vi "Bin to BDC(5-разрядное число).vi"(0 "B":T2) -> (1 "R0":T1, 2 "R1":T1)   [LabVIEW 2013]
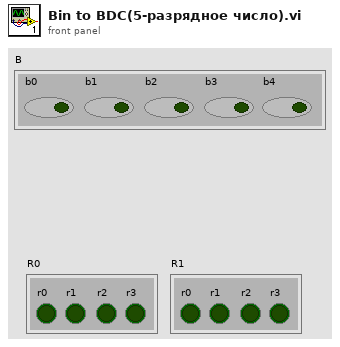
[diagram p1: front panel]
types:
  T1 = cluster{"r0":bool, "r1":bool, "r2":bool, "r3":bool}
  T2 = cluster{"b0":bool, "b1":bool, "b2":bool, "b3":bool, "b4":bool}
  T3 = cluster{"r0":bool, "r1":bool, "r2":bool, "r3":bool, "r4":bool}
  T4 = cluster{"r1":bool, "r2":bool, "r3":bool, "r4":bool}
  T5 = cluster{"d0":bool, "d1":bool, "d2":bool, "d3":bool}
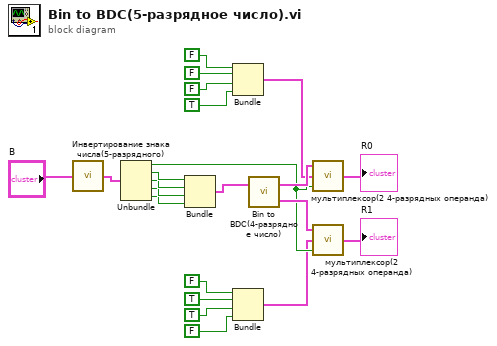
[diagram p0: block diagram]
diagram:
  n1 = call "Инвертирование знака числа(5-разрядного).vi"("A"="B") -> ("R"=w2:T3)
  n2 = Unbundle(w2) -> ("r0"=w13:bool, "r1"=w22:bool, "r2"=w21:bool, "r3"=w20:bool, "r4"=w19:bool)
  n3 = Bundle("r1"=w22, "r2"=w21, "r3"=w20, "r4"=w19) -> (w18:T4)  [unwired: 1 in]
  n4 = Bundle(FALSE, FALSE, FALSE, TRUE) -> (w8:cluster{bool, bool, bool, bool})  [unwired: 1 in]
  n5 = Bundle(FALSE, TRUE, TRUE, FALSE) -> (w3:cluster{bool, bool, bool, bool})  [unwired: 1 in]
  n6 = call "Bin to BDC(4-разрядное число).vi"("B"=w18) -> ("D1"=w15:T5, "D0"=w14:T5)  [unwired: 1 in]
  n7 = call "мультиплексор(2 4-разрядных операнда).vi"("c"=w13, "B"=w8, "A"=w14) -> ("R"=→"R0":T1)
  n8 = call "мультиплексор(2 4-разрядных операнда).vi"("c"=w13, "B"=w3, "A"=w15) -> ("R"=→"R1":T1)
